vi "WPI_DashboardNew Image Display Size.vi"(10 "NewBnds":T1, 11 "Size Constraints":cluster{"min tab width":i32, "w/h":dbl}) -> (0 "Window Width":i16, 1 "Window Height":i16, 2 "Height":dbl, 3 "Width":dbl)   [LabVIEW 2017]
uses:
  <vilib>/Utility/miscctls.llb/LVRectTypeDef.ctl
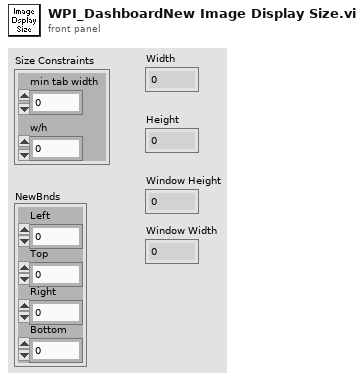
[diagram p1: front panel]
types:
  T1 = typedef "LVRectTypeDef.ctl" = cluster{"Left":i16, "Top":i16, "Right":i16, "Bottom":i16}
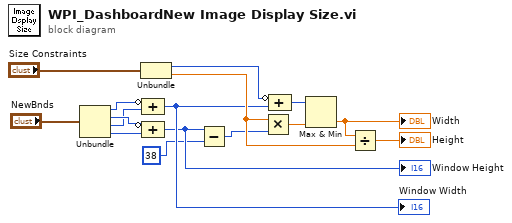
[diagram p0: block diagram]
diagram:
  n1 = Unbundle("NewBnds") -> ("Left"=w8:i16, "Top"=w16:i16, "Right"=w7:i16, "Bottom"=w6:i16)
  n2 = Unbundle("Size Constraints") -> ("min tab width"=w10:i32, "w/h"=w13:dbl)
  n3 = Compound Arithmetic op=ADD(invert w8, w7) -> (w4:i16)
  "Window Width" <- w4
  n4 = Compound Arithmetic op=ADD(invert w16, w6) -> (w3:i16)
  "Window Height" <- w3
  n5 = Subtract(x=w3, y=38) -> (x-y=w2:i32)
  n6 = Multiply(x=w13, y=w2) -> (x*y=w12:dbl)
  n7 = Compound Arithmetic op=ADD(invert w10, w4) -> (w11:i32)
  n8 = Max & Min(x=w11, y=w12) -> (min(x,y)=w14:dbl)  [unwired: 1 out]
  "Width" <- w14
  n9 = Divide(x=w14, y=w13) -> (x/y=→"Height":dbl)
